vi "imp_test_v9_3.vi"() -> ()   [LabVIEW 2014]
uses:
  <vilib>/rvi/FXPMathLib/FxpSinAndCos/subVIs/nifxpmath_SinAndCos_SimConfig.ctl
  <vilib>/rvi/Emulation/niFpgaGetClockAttributes.vi
  <vilib>/rvi/Emulation/niFpgaSctlEmulationGetInTimedLoop.vi
  <vilib>/rvi/Emulation/niFpgaEmulationReportErrorSimple.vi
  <vilib>/rvi/Emulation/niFpgaProcessEmulError.vi
  <vilib>/rvi/interface/RandomDataEmulation/nirviRandomDataMultiElementFPGAFIFO.vi
  <instcachedir>/0/nirviRandomDataMultiElementFPGAFIFO_AD0CFC12EF974623A9C2E4184BC062B2.lvgen/nirviRandomDataMultiElementFPGAFIFO_AD0CFC12EF974623A9C2E4184BC062B2_025.vi
  <vilib>/rvi/interface/RandomDataEmulation/niFpgaRandomDataHandleErrors.vi
  <vilib>/rvi/Emulation/niFpgaCriticalErrorInLSC.vi
  <vilib>/rvi/FXPMathLib/FxpSinAndCos/simVIs/DllFxpSinAndCosTemp_sub.vi
  <vilib>/rvi/eio/common/nirviEmuTemplateMethod_errors.vi
  <vilib>/rvi/DataTransferAndStorage/Container/XNode/niFpgaContainer.xnode
  <vilib>/rvi/interface/RandomDataEmulation/nirviRandomDataFpgaMultiElementTemplate.vi
  <vilib>/rvi/FXPMathLib/FxpSinAndCos/XNode/nifxpmath_SinAndCos.xnode
  <vilib>/eio/EIONode/EIONode.xnode
  <vilib>/rvi/Analysis/measure/butterworth/XNode/niFpgaButterworthFilter.xnode
panel:
  out "Dpr_ramp":fxp<+/-,22,7>
  out "Dyr_ramp":fxp<+/-,22,7>
  in  "Dp_stroke (mm)":fxp<+/-,22,7>
  in  "Dy_stroke (mm)":fxp<+/-,22,7>
  in  "Vp (mm/s)":fxp<+/-,30,6>
  in  "Vy (mm/s)":fxp<+/-,30,6>
  out "omega_p (Mavg w. f)":fxp<+/-,36,18>
  in  "scaled coefficients":i32[](array[numeric])=[946630756, 63555534]
  in  "FIFO":i16(ring) items=["Pitch_F+P", "imp ctrl", "Yaw_F+P"]
  out "PID (kHz)":fxp<+/-,20,10>
  out "Dy1_d (T)":fxp<+/-,36,13>
  out "omega_y1 (T)":fxp<+/-,36,13>
  out "Dp1_d (T)":fxp<+/-,36,13>
  out "omega_p1 (T)":fxp<+/-,36,13>
  out "Dy2_d (T)":fxp<+/-,36,13>
  out "Dp2_d (T)":fxp<+/-,36,13>
  out "omega_y2 (T)":fxp<+/-,36,13>
  out "omega_p2 (T)":fxp<+/-,36,13>
  out "mt_omega_y2":u32
  out "mt_omega_p2":u32
  out "rad_y2":fxp<+/-,33,20>
  out "D_y2":fxp<+/-,32,7>
  out "rad_y1":fxp<+/-,33,20>
  out "D_y1":fxp<+/-,32,7>
  out "Encoder Position_y1":i32
  out "Encoder Position_y2":i32
  out "Encoder Position_p2":i32
  out "D_p2":fxp<+/-,32,7>
  out "rad_p2":fxp<+/-,33,20>
  out "D_p1":fxp<+/-,32,7>
  out "rad_p1":fxp<+/-,33,20>
  out "Encoder Position_p1":i32
  in  "Mag. factor_y":fxp<+/-,20,3>
  in  "Mag. encoder_y":bool
  out "omega_y (rad/s)":fxp<+/-,36,13>
  out "Dy_d (mm/s)":fxp<+/-,36,13>
  in  "Vy. Est.":i16(ring) items=["T", "Mavg"]
  out "omega_y (Mavg)":fxp<+/-,36,14>
  out "Dy_d (Mavg)":fxp<+/-,36,14>
  in  "Dy_d_M_avg_Tc (uSec)":i32
  out "Dp_d (Mavg)":fxp<+/-,36,14>
  out "omega_p (Mavg)":fxp<+/-,36,14>
  in  "Dp_d_M_avg_Tc (uSec)":i32
  out "Dp_d (T)":fxp<+/-,36,13>
  out "omega_p (T)":fxp<+/-,36,13>
  in  "Vp. Est.":i16(ring) items=["T", "Mavg"]
  in  "Mag. factor_p":fxp<+/-,20,3>
  in  "Mag. encoder_p":bool
  in  "Belt_out_p":fxp<+/-,7,7>
  in  "Belt_in_p":fxp<+/-,6,6>
  in  "Belt_out_y":fxp<+/-,7,7>
  in  "Belt_in_y":fxp<+/-,6,6>
  in  "mt0_omega_p":u32
  in  "Encoder reset":bool
  out "Dpr_sin":fxp<+/-,22,7>
  in  "Sin offset_p":fxp<+/-,22,7>
  in  "Sin magnitude_p":fxp<+/-,21,6>
  out "Dpr_sin_dd":fxp<+/-,35,20>
  out "Dpr_sin_d":fxp<+/-,33,15>
  out "Sin omega_p":fxp<+/-,34,9>
  in  "Sin wave freq._p (Hz)":fxp<+/-,32,6>
  in  "Dpr_step":fxp<+/-,22,7>
  out "Dpr_for":fxp<+/-,22,7>
  in  "Command_p":i16(ring) items=["Step", "Sine", "Ramp"]
  out "Fp_PID":fxp<+/-,36,16>
  in  "Kp_p":fxp<+/-,32,13>
  out "va_p":fxp<+/-,36,7>
  out "vb_p":fxp<+/-,37,8>
  out "vq_p_F":fxp<+/-,20,5> format="%.57g"
  out "vd_p_F":fxp<+/-,20,5>
  in  "Stop motor_p":bool
  out "Dp_d (mm/s)":fxp<+/-,36,13>
  out "omega_p (rad/s)":fxp<+/-,36,13>
  out "mt_omega_p1":u32
  out "rad_p(NrTheta)":fxp<+/-,33,20>
  out "D_p(mm)":fxp<+/-,32,7>
  out "Encoder Position_p":i32
  in  "Encoder reset_p":bool
  out "Dyr_for":fxp<+/-,22,7>
  in  "Command_y":i16(ring) items=["Step", "Sine", "Ramp"]
  out "vb_y":fxp<+/-,38,8>
  out "va_y":fxp<+/-,38,8>
  out "Dyr_sin_dd":fxp<+/-,35,20>
  out "Dyr_sin_d":fxp<+/-,33,15>
  out "Sin omega_y":fxp<+/-,34,9>
  out "Dyr_sin":fxp<+/-,22,7>
  in  "Sin offset_y":fxp<+/-,22,7>
  in  "Sin magnitude_y":fxp<+/-,21,6>
  out "Time now(s)":fxp<+,52,14>
  in  "Sin wave freq._y (Hz)":fxp<+/-,32,6>
  in  "Dyr_step":fxp<+/-,22,7>
  out "Fy_PID":fxp<+/-,36,16>
  in  "Kp_y":fxp<+/-,32,13>
  out "vq_y_F":fxp<+/-,20,5> format="%.57g"
  out "vd_y_F":fxp<+/-,20,5>
  in  "Stop motor_y":bool
  out "Dy_d (T)":fxp<+/-,36,13>
  out "omega_y (T)":fxp<+/-,36,13>
  in  "mt0_omega_y":u32
  out "mt_omega_y1":u32
  out "rad_y(NrTheta)":fxp<+/-,33,20>
  out "D_y(mm)":fxp<+/-,32,7>
  out "Encoder Position_y":i32
  in  "Encoder reset_y":bool
  in  "Ini coe.":bool
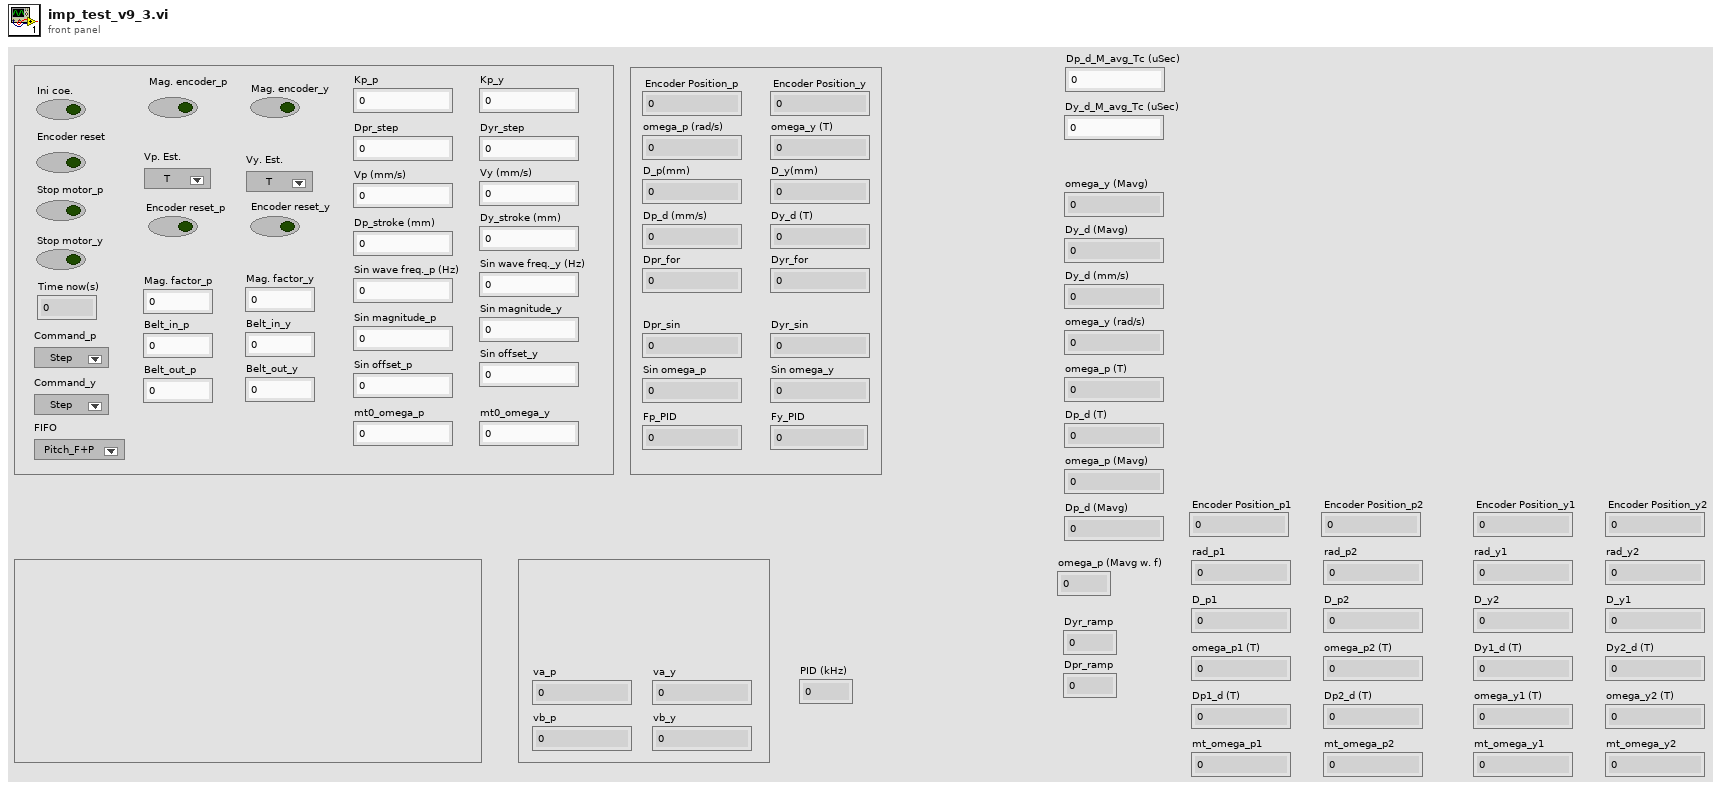
[diagram p1: front panel]
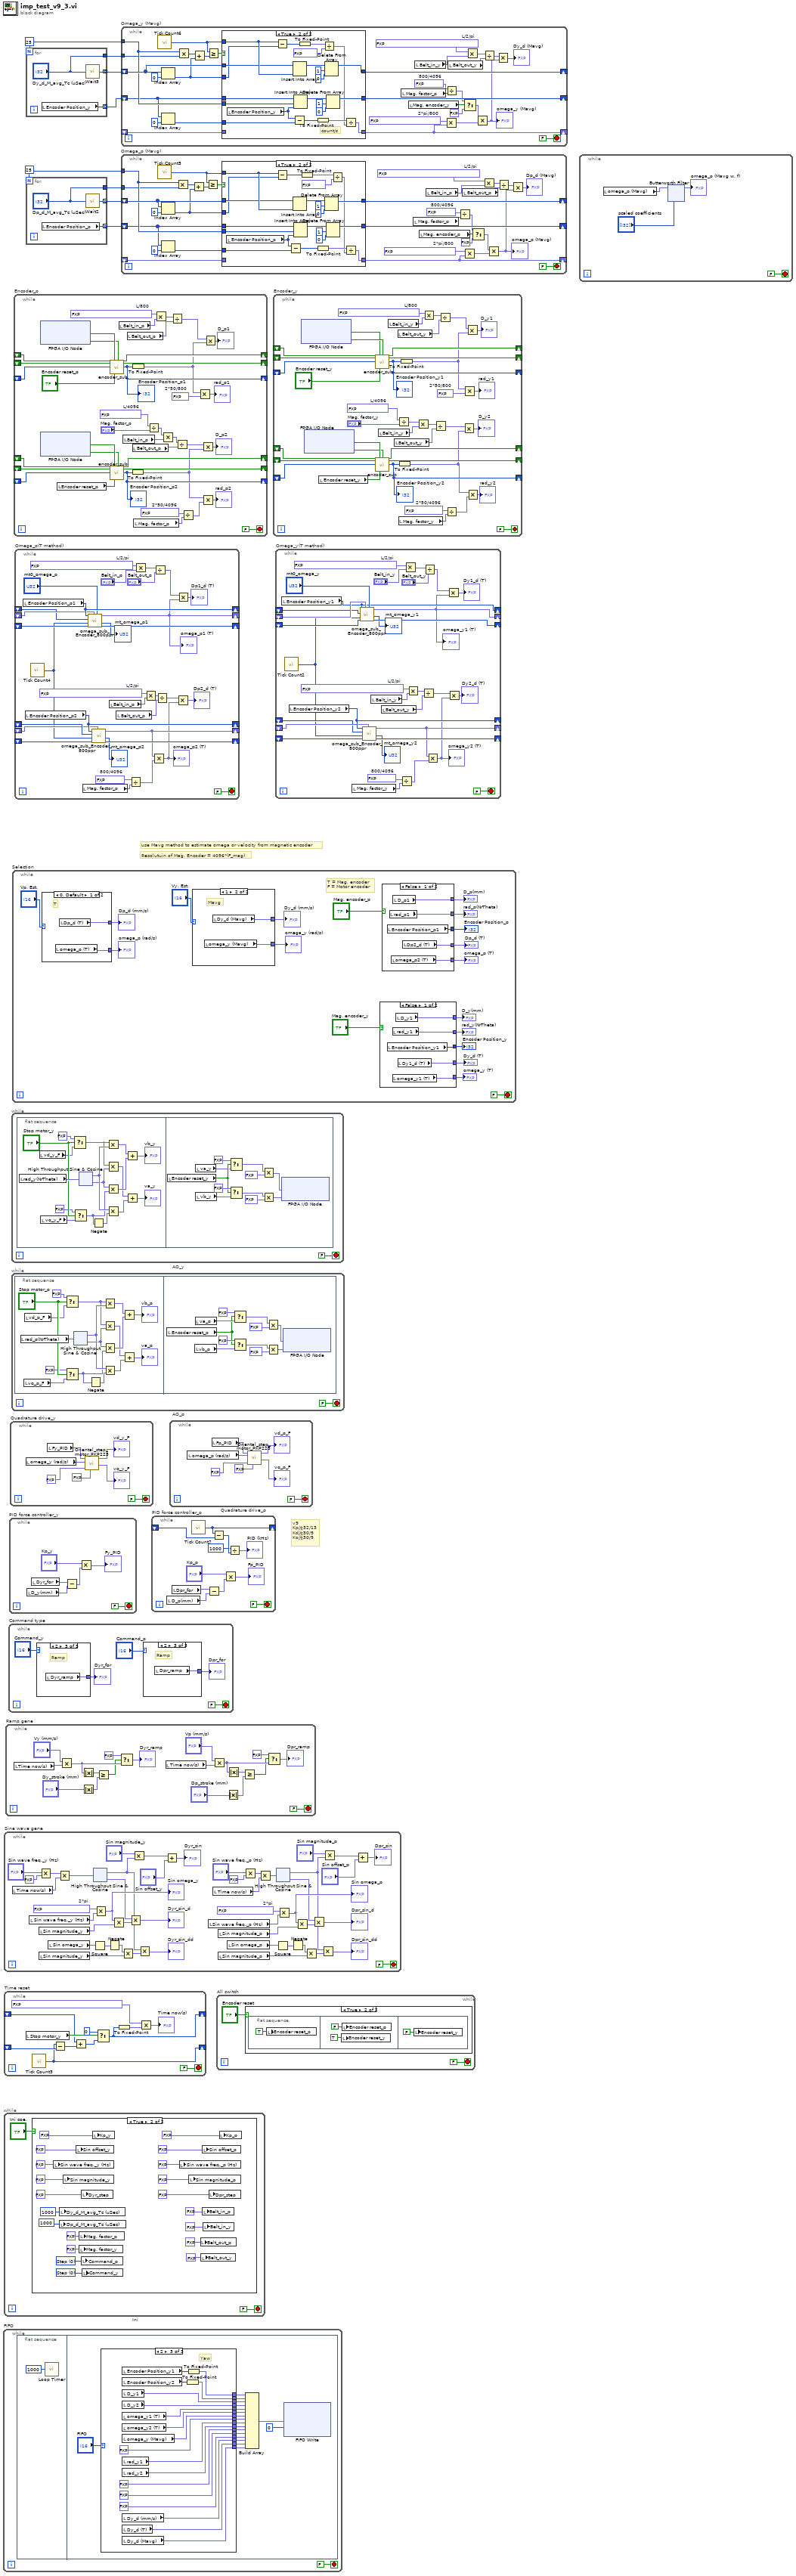
[diagram p0: block diagram]
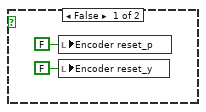
[diagram p4: hidden frame]
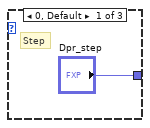
[diagram p5: hidden frame]
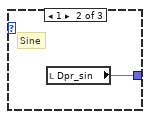
[diagram p6: hidden frame]
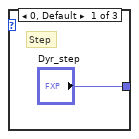
[diagram p7: hidden frame]
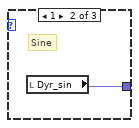
[diagram p8: hidden frame]
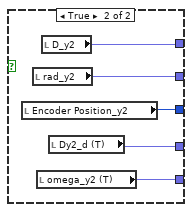
[diagram p9: hidden frame]
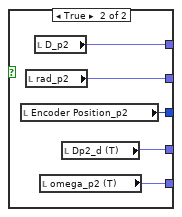
[diagram p10: hidden frame]
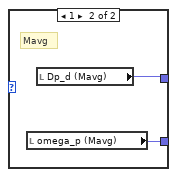
[diagram p11: hidden frame]
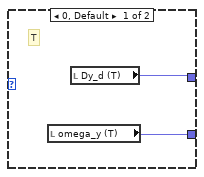
[diagram p12: hidden frame]
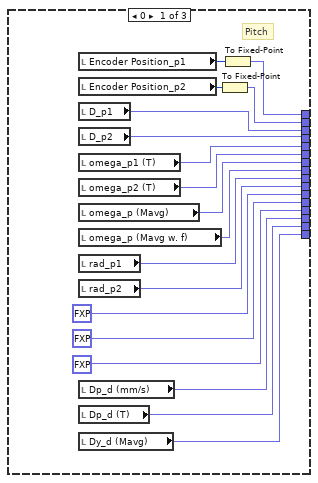
[diagram p14: hidden frame]
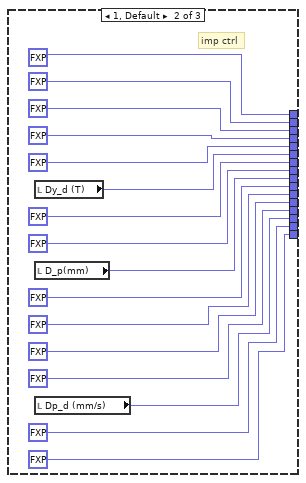
[diagram p15: hidden frame]
diagram:
  w5 = 25
  w8 = 25
  # "v9\nKp改32/13\nKd改30/9\nKo改30/9"
  # "Resolutuin of Mag. Encoder = 4096*(F_mag)"
  # "use Mavg method to estimate omega or velocity from magnetic encoder"
  n1 = while "FIFO" {
    stop <- FALSE stop-if-true
    n2 = flat-sequence {
      frame #0 {
        n3 = call "Loop Timer"("Count(uSec)"=u32 1000) -> ()  [unwired: 1 out]
      }
      frame #1 {
        n4 = case shown="2" "FIFO" {
          tunnel: [w30 fxp<+,1,1> 0.0 w64] -> w11
          tunnel: [w31 fxp<+,1,1> 0.0 w65] -> w29
          tunnel: [w47 fxp<+,1,1> 0.0 w81] -> w28
          tunnel: [w46 fxp<+,1,1> 0.0 w80] -> w27
          tunnel: [w43 fxp<+,1,1> 0.0 w77] -> w25
          tunnel: [w44 w63 w78] -> w24
          tunnel: [w45 fxp<+,1,1> 0.0 w79] -> w23
          tunnel: [w42 w62 w76] -> w22
          tunnel: [w41 fxp<+,1,1> 0.0 w75] -> w21
          tunnel: [fxp<+,1,1> 0.0 fxp<+,1,1> 0.0 fxp<+,1,1> 0.0] -> w20
          tunnel: [fxp<+,1,1> 0.0 fxp<+,1,1> 0.0 fxp<+,1,1> 0.0] -> w19
          tunnel: [fxp<+,1,1> 0.0 fxp<+,1,1> 0.0 fxp<+,1,1> 0.0] -> w18
          tunnel: [w40 w61 w74] -> w17
          tunnel: [w39 fxp<+,1,1> 0.0 w73] -> w16
          tunnel: [w34 fxp<+,1,1> 0.0 ("element") w72] -> w15
          tunnel: [w38 fxp<+,1,1> 0.0 fxp<+,1,1> 0.0] -> w13
          frame 0 {
            # "Pitch"
            n5 = local read "Encoder Position_p1"() -> (w33:i32)
            n6 = local read "Encoder Position_p2"() -> (w32:i32)
            n7 = local read "D_p1"() -> (w47:fxp<+/-,32,7>)
            n8 = local read "D_p2"() -> (w46:fxp<+/-,32,7>)
            n9 = local read "omega_p1 (T)"() -> (w45:fxp<+/-,36,13>)
            n10 = local read "omega_p2 (T)"() -> (w44:fxp<+/-,36,13>)
            n11 = local read "omega_p (Mavg)"() -> (w43:fxp<+/-,36,14>)
            n12 = local read "omega_p (Mavg w. f)"() -> (w38:fxp<+/-,36,18>)
            n13 = local read "rad_p1"() -> (w42:fxp<+/-,33,20>)
            n14 = local read "rad_p2"() -> (w41:fxp<+/-,33,20>)
            n15 = local read "Dp_d (mm/s)"() -> (w40:fxp<+/-,36,13>)
            n16 = local read "Dp_d (T)"() -> (w39:fxp<+/-,36,13>)
            n17 = local read "Dy_d (Mavg)"() -> (w34:fxp<+/-,36,14>)
            n18 = To Fixed-Point(number=w32) -> (fixed-point=w31:fxp<+/-,25,25>)  [unwired: 1 in]
            n19 = To Fixed-Point(number=w33) -> (fixed-point=w30:fxp<+/-,25,25>)  [unwired: 1 in]
          }
          frame 1, Default {
            # "imp ctrl"
            n20 = local read "Dy_d (T)"() -> (w63:fxp<+/-,36,13>)
            n21 = local read "D_p(mm)"() -> (w62:fxp<+/-,32,7>)
            n22 = local read "Dp_d (mm/s)"() -> (w61:fxp<+/-,36,13>)
          }
          frame 2 {
            # "Yaw"
            n23 = local read "Encoder Position_y1"() -> (w67:i32)
            n24 = local read "Encoder Position_y2"() -> (w66:i32)
            n25 = local read "D_y1"() -> (w81:fxp<+/-,32,7>)
            n26 = local read "D_y2"() -> (w80:fxp<+/-,32,7>)
            n27 = local read "omega_y1 (T)"() -> (w79:fxp<+/-,36,13>)
            n28 = local read "omega_y2 (T)"() -> (w78:fxp<+/-,36,13>)
            n29 = local read "omega_y (Mavg)"() -> (w77:fxp<+/-,36,14>)
            n30 = local read "rad_y1"() -> (w76:fxp<+/-,33,20>)
            n31 = local read "rad_y2"() -> (w75:fxp<+/-,33,20>)
            n32 = local read "Dy_d (mm/s)"() -> (w74:fxp<+/-,36,13>)
            n33 = local read "Dy_d (T)"() -> (w73:fxp<+/-,36,13>)
            n34 = local read "Dy_d (Mavg)"() -> (w72:fxp<+/-,36,14>)
            n35 = To Fixed-Point(number=w66) -> (fixed-point=w65:fxp<+/-,25,25>)  [unwired: 1 in]
            n36 = To Fixed-Point(number=w67) -> (fixed-point=w64:fxp<+/-,25,25>)  [unwired: 1 in]
          }
        }
        n37 = Build Array(w11, w29, w28, w27, w23, w24, w25, w13, w22, w21, w20, w19, w18, w17, w16, w15) -> (w14:fxp<+/-,50,25>[])
        n38 = xnode ("FIFO Write")("Element"=w14, "Timeout"=0) -> ()  [unwired: 1 in, 2 out]
      }
    }
  }
  n39 = while "Sine wave gene" {
    stop <- FALSE stop-if-true
    w87 = fxp<+,20,3> 6.2831878662109375  # 2*pi
    w119 = fxp<+,20,3> 6.2831878662109375  # 2*pi
    n40 = local read "Time now(s)"() -> (w125:fxp<+,52,14>)
    n41 = local read "Sin wave freq._y (Hz)"() -> (w118:fxp<+/-,32,6>)
    n42 = Multiply(x="Sin wave freq._y (Hz)", y=fxp<+/-,10,3> 2.0) -> (x*y=w126:fxp<+/-,41,9>)
    n43 = local read "Sin magnitude_y"() -> (w116:fxp<+/-,21,6>)
    n44 = local read "Sin magnitude_y"() -> (w109:fxp<+/-,21,6>)
    n45 = local read "Sin omega_y"() -> (w112:fxp<+/-,34,9>)
    n46 = Multiply(x=w126, y=w125) -> (x*y=w124:fxp<+/-,41,19>)
    n47 = Square(x=w112) -> (x^2=w111:fxp<+,34,18>)
    n48 = xnode "High Throughput Sine & Cosine"("x (pi)"=w124) -> ("sin(x)"=w106:fxp<+/-,16,2>, "cos(x)"=w114:fxp<+/-,16,2>)
    n49 = Multiply(x=w119, y=w118) -> (x*y=w117:fxp<+/-,34,9>)
    "Sin omega_y" <- w117
    n50 = Negate(x=w111) -> (-x=w110:fxp<+/-,35,19>)
    n51 = Multiply(x=w117, y=w116) -> (x*y=w115:fxp<+/-,33,15>)
    n52 = Multiply(x=w110, y=w109) -> (x*y=w108:fxp<+/-,34,20>)
    n53 = Multiply(x=w114, y=w115) -> (x*y=→"Dyr_sin_d":fxp<+/-,33,15>)
    n54 = Multiply(x="Sin magnitude_y", y=w106) -> (x*y=w122:fxp<+/-,37,8>)
    n55 = Multiply(x=w106, y=w108) -> (x*y=→"Dyr_sin_dd":fxp<+/-,35,20>)
    n56 = Add(x=w122, y="Sin offset_y") -> (x+y=→"Dyr_sin":fxp<+/-,37,8>)
    n57 = local read "Sin wave freq._p (Hz)"() -> (w83:fxp<+/-,32,6>)
    n58 = local read "Time now(s)"() -> (w101:fxp<+,52,14>)
    n59 = local read "Sin magnitude_p"() -> (w84:fxp<+/-,21,6>)
    n60 = local read "Sin magnitude_p"() -> (w86:fxp<+/-,21,6>)
    n61 = local read "Sin omega_p"() -> (w85:fxp<+/-,34,9>)
    n62 = Multiply(x="Sin wave freq._p (Hz)", y=fxp<+/-,10,3> 2.0) -> (x*y=w105:fxp<+/-,42,9>)
    n63 = Multiply(x=w105, y=w101) -> (x*y=w102:fxp<+/-,41,19>)
    n64 = Square(x=w85) -> (x^2=w97:fxp<+,34,18>)
    n65 = xnode "High Throughput Sine & Cosine"("x (pi)"=w102) -> ("sin(x)"=w88:fxp<+/-,16,2>, "cos(x)"=w93:fxp<+/-,16,2>)
    n66 = Multiply(x=w87, y=w83) -> (x*y=w100:fxp<+/-,34,9>)
    "Sin omega_p" <- w100
    n67 = Negate(x=w97) -> (-x=w96:fxp<+/-,35,19>)
    n68 = Multiply(x=w100, y=w84) -> (x*y=w99:fxp<+/-,33,15>)
    n69 = Multiply(x=w96, y=w86) -> (x*y=w95:fxp<+/-,35,19>)
    n70 = Multiply(x=w93, y=w99) -> (x*y=→"Dpr_sin_d":fxp<+/-,33,15>)
    n71 = Multiply(x=w88, y=w95) -> (x*y=→"Dpr_sin_dd":fxp<+/-,35,20>)
    n72 = Multiply(x="Sin magnitude_p", y=w88) -> (x*y=w91:fxp<+/-,37,8>)
    n73 = Add(x=w91, y="Sin offset_p") -> (x+y=→"Dpr_sin":fxp<+/-,37,8>)
  }
  n74 = while "Time reset" {
    shift-right: [w198] -> _
    shift-left: _ -> [w199]
    shift-right: [w193] -> _
    shift-left: _ -> [w194]
    stop <- FALSE stop-if-true
    n75 = local read "Stop motor_y"() -> (w200:bool)
    n76 = call "Tick Count3"() -> ("Tick Count(uSec)"=w198:u32)
    n77 = Subtract(x=w198, y=w199) -> (x-y=w197:u32)
    n78 = Add(x=w194, y=w197) -> (x+y=w196:u32)
    n79 = Select(t=u32 0, s=w200, f=w196) -> (s? t:f=w193:u32)
    n80 = To Fixed-Point(number=w193) -> (fixed-point=w192:fxp<+,32,32>)  [unwired: 1 in]
    n81 = Multiply(x=fxp<+,20,-18> 1.0000003385357559e-06, y=w192) -> (x*y=→"Time now(s)":fxp<+,52,14>)
  }
  n82 = while "Ini" {
    stop <- FALSE stop-if-true
    n83 = case shown="True" "Ini coe." {
      frame False {
      }
      frame True {
        w216 = i16 0 items=["Step", "Sine"] ("Command_p")
        w217 = i16 0 items=["Step", "Sine"] ("Command_y")
        n84 = local write "Sin wave freq._y (Hz)"(fxp<+/-,32,6> 1.0 ("Sin wave freq. (Hz)")) -> ()
        n85 = local write "Dp_d_M_avg_Tc (uSec)"(u32 1000 ("D_d_M_avg_Tc (uSec)")) -> ()
        n86 = local write "Dy_d_M_avg_Tc (uSec)"(1000 ("Dy_d_M_avg_Tc (uSec)")) -> ()
        n87 = local write "Sin magnitude_y"(fxp<+/-,22,7> 5.0 ("Sin magnitude")) -> ()
        n88 = local write "Sin offset_y"(fxp<+/-,38,9> 0.0 ("Sin offset")) -> ()
        n89 = local write "Mag. factor_p"(fxp<+/-,20,3> 1.0 ("Mag. factor_p")) -> ()
        n90 = local write "Mag. factor_y"(fxp<+/-,20,3> 1.0 ("Mag. factor_y")) -> ()
        n91 = local write "Command_p"(w216) -> ()
        n92 = local write "Dyr_step"(fxp<+/-,22,7> 0.0 ("Dr")) -> ()
        n93 = local write "Command_y"(w217) -> ()
        n94 = local write "Kp_y"(fxp<+/-,36,9> 30.0 ("Kp")) -> ()
        n95 = local write "Sin wave freq._p (Hz)"(fxp<+/-,32,6> 1.0 ("Sin wave freq._p (Hz)")) -> ()
        n96 = local write "Sin magnitude_p"(fxp<+/-,21,6> 5.0 ("Sin magnitude_p")) -> ()
        n97 = local write "Belt_out_p"(fxp<+/-,7,7> 22.0 ("Belt_op")) -> ()
        n98 = local write "Belt_out_y"(fxp<+/-,7,7> 22.0 ("Belt_oy")) -> ()
        n99 = local write "Sin offset_p"(fxp<+/-,22,7> 0.0 ("Sin offset_p")) -> ()
        n100 = local write "Belt_in_p"(fxp<+/-,6,6> 16.0 ("Belt_mp")) -> ()
        n101 = local write "Belt_in_y"(fxp<+/-,6,6> 16.0 ("Belt_my")) -> ()
        n102 = local write "Dpr_step"(fxp<+/-,22,7> 0.0 ("Dpr_step")) -> ()
        n103 = local write "Kp_p"(fxp<+/-,36,9> 30.0 ("Kp_p")) -> ()
      }
    }
  }
  n104 = while "Ramp gene" {
    stop <- FALSE stop-if-true
    n105 = local read "Time now(s)"() -> (w240:fxp<+,52,14>)
    n106 = Multiply(x="Vy (mm/s)", y=w240) -> (x*y=w229:fxp<+/-,64,20>)
    n107 = Absolute Value(x=w229) -> (abs(x)=w237:fxp<+,64,20>)
    n108 = Absolute Value(x="Dy_stroke (mm)") -> (abs(x)=w236:fxp<+,22,7>)
    n109 = Greater Or Equal?(x=w237, y=w236) -> (x >= y?=w228:bool)
    n110 = Select(t=fxp<+,1,1> 0.0, s=w228, f=w229) -> (s? t:f=→"Dyr_ramp":fxp<+/-,64,20>)
    n111 = local read "Time now(s)"() -> (w238:fxp<+,52,14>)
    n112 = Multiply(x="Vp (mm/s)", y=w238) -> (x*y=w227:fxp<+/-,64,20>)
    n113 = Absolute Value(x="Dp_stroke (mm)") -> (abs(x)=w233:fxp<+,22,7>)
    n114 = Absolute Value(x=w227) -> (abs(x)=w234:fxp<+,64,20>)
    n115 = Greater Or Equal?(x=w234, y=w233) -> (x >= y?=w226:bool)
    n116 = Select(t=fxp<+,1,1> 0.0, s=w226, f=w227) -> (s? t:f=→"Dpr_ramp":fxp<+/-,64,20>)
  }
  n117 = while "Command type" {
    stop <- FALSE stop-if-true
    n118 = case shown="2" "Command_y" {
      tunnel: ["Dyr_step" w251 w252] -> w245
      frame 0, Default {
        # "Step"
      }
      frame 1 {
        # "Sine"
        n119 = local read "Dyr_sin"() -> (w251:fxp<+/-,22,7>)
      }
      frame 2 {
        # "Ramp"
        n120 = local read "Dyr_ramp"() -> (w252:fxp<+/-,22,7>)
      }
    }
    "Dyr_for" <- w245
    n121 = case shown="2" "Command_p" {
      tunnel: ["Dpr_step" w248 w249] -> w243
      frame 0, Default {
        # "Step"
      }
      frame 1 {
        # "Sine"
        n122 = local read "Dpr_sin"() -> (w248:fxp<+/-,22,7>)
      }
      frame 2 {
        # "Ramp"
        n123 = local read "Dpr_ramp"() -> (w249:fxp<+/-,22,7>)
      }
    }
    "Dpr_for" <- w243
  }
  n124 = while "PID force controller_y" {
    stop <- FALSE stop-if-true
    n125 = local read "D_y(mm)"() -> (w256:fxp<+/-,32,7>)
    n126 = local read "Dyr_for"() -> (w257:fxp<+/-,22,7>)
    n127 = Subtract(x=w257, y=w256) -> (x-y=w255:fxp<+/-,33,8>)
    n128 = Multiply(x="Kp_y", y=w255) -> (x*y=→"Fy_PID":fxp<+/-,64,20>)
  }
  n129 = while "Quadrature drive_y" {
    stop <- FALSE stop-if-true
    n130 = local read "omega_y (rad/s)"() -> (w265:fxp<+/-,36,13>)
    n131 = local read "Fy_PID"() -> (w261:fxp<+/-,36,16>)
    n132 = call "Oriental_step_motor_PKP225.vi"("F_Threshold"=fxp<+,12,12> 10.0, "dFmr"=fxp<+,1,1> 0.0 ("f"), "omega"=w265, "Fmr"=w261) -> ("vq_F"=→"vq_y_F":fxp<+/-,20,5>, "vd_F"=→"vd_y_F":fxp<+/-,20,5>)  [unwired: 6 in]
  }
  n133 = while "AO_p" {
    stop <- FALSE stop-if-true
    n134 = flat-sequence {
      frame #0 {
        n135 = local read "rad_p(NrTheta)"() -> (w278:fxp<+/-,33,20>)
        n136 = local read "vq_p_F"() -> (w279:fxp<+/-,20,5>)
        n137 = local read "vd_p_F"() -> (w281:fxp<+/-,20,5>)
        n138 = Select(t=fxp<+/-,20,5> 0.0, s="Stop motor_p", f=w281) -> (s? t:f=w270:fxp<+/-,20,5>)
        n139 = Select(t=fxp<+,1,1> 0.0, s="Stop motor_p", f=w279) -> (s? t:f=w269:fxp<+/-,20,5>)
        n140 = xnode "High Throughput Sine & Cosine"("x (pi)"=w278) -> ("sin(x)"=w272:fxp<+/-,16,2>, "cos(x)"=w271:fxp<+/-,16,2>)
        n141 = Negate(x=w269) -> (-x=w277:fxp<+/-,21,6>)
        n142 = Multiply(x=w270, y=w272) -> (x*y=w276:fxp<+/-,36,7>)
        n143 = Multiply(x=w270, y=w271) -> (x*y=w274:fxp<+/-,36,7>)
        n144 = Multiply(x=w271, y=w269) -> (x*y=w275:fxp<+/-,36,7>)
        n145 = Multiply(x=w272, y=w277) -> (x*y=w273:fxp<+/-,35,6>)
        n146 = Add(x=w276, y=w275) -> (x+y=→"vb_p":fxp<+/-,37,8>)
        n147 = Add(x=w274, y=w273) -> (x+y=→"va_p":fxp<+/-,36,7>)
      }
      frame #1 {
        n148 = local read "Encoder reset_p"() -> (w314:bool)
        n149 = local read "vb_p"() -> (w315:fxp<+/-,37,8>)
        n150 = local read "va_p"() -> (w316:fxp<+/-,36,7>)
        n151 = Select(t=fxp<+,2,2> 3.0, s=w314, f=w316) -> (s? t:f=w322:fxp<+/-,36,7>)
        n152 = Select(t=fxp<+,1,1> 0.0, s=w314, f=w315) -> (s? t:f=w321:fxp<+/-,37,8>)
        n153 = Multiply(x=w322, y=fxp<+/-,1,0> -0.5) -> (x*y=w317:fxp<+/-,36,6>)
        n154 = Multiply(x=w321, y=fxp<+/-,1,0> -0.5) -> (x*y=w318:fxp<+/-,36,6>)
        n155 = xnode "FPGA I/O Node"("Mod8/AO0"=w317, "Mod8/AO1"=w318) -> ()  [unwired: 2 in, 2 out]
      }
    }
  }
  n156 = while "AO_y" {
    stop <- FALSE stop-if-true
    n157 = flat-sequence {
      frame #0 {
        n158 = local read "rad_y(NrTheta)"() -> (w342:fxp<+/-,33,20>)
        n159 = local read "vd_y_F"() -> (w340:fxp<+/-,20,5>)
        n160 = local read "vq_y_F"() -> (w339:fxp<+/-,20,5>)
        n161 = Select(t=fxp<+/-,20,5> 0.0, s="Stop motor_y", f=w340) -> (s? t:f=w334:fxp<+/-,20,5>)
        n162 = Select(t=fxp<+/-,20,5> 0.0, s="Stop motor_y", f=w339) -> (s? t:f=w333:fxp<+/-,20,5>)
        n163 = xnode "High Throughput Sine & Cosine"("x (pi)"=w342) -> ("sin(x)"=w336:fxp<+/-,17,2>, "cos(x)"=w335:fxp<+/-,17,2>)
        n164 = Negate(x=w333) -> (-x=w332:fxp<+/-,21,6>)
        n165 = Multiply(x=w334, y=w336) -> (x*y=w331:fxp<+/-,37,7>)
        n166 = Multiply(x=w334, y=w335) -> (x*y=w329:fxp<+/-,37,7>)
        n167 = Multiply(x=w335, y=w333) -> (x*y=w330:fxp<+/-,37,7>)
        n168 = Multiply(x=w336, y=w332) -> (x*y=w328:fxp<+/-,36,6>)
        n169 = Add(x=w331, y=w330) -> (x+y=→"vb_y":fxp<+/-,38,8>)
        n170 = Add(x=w329, y=w328) -> (x+y=→"va_y":fxp<+/-,37,7>)
      }
      frame #1 {
        n171 = local read "Encoder reset_y"() -> (w375:bool)
        n172 = local read "va_y"() -> (w374:fxp<+/-,38,8>)
        n173 = local read "vb_y"() -> (w373:fxp<+/-,38,8>)
        n174 = Select(t=fxp<+,2,2> 3.0, s=w375, f=w374) -> (s? t:f=w379:fxp<+/-,38,8>)
        n175 = Select(t=fxp<+,1,1> 0.0, s=w375, f=w373) -> (s? t:f=w378:fxp<+/-,38,8>)
        n176 = Multiply(x=w379, y=fxp<+/-,1,0> -0.5) -> (x*y=w382:fxp<+/-,39,8>)
        n177 = Multiply(x=w378, y=fxp<+/-,1,0> -0.5) -> (x*y=w383:fxp<+/-,37,6>)
        n178 = xnode "FPGA I/O Node"("Mod8/AO2"=w382, "Mod8/AO3"=w383) -> ()  [unwired: 2 in, 2 out]
      }
    }
  }
  n179 = while "Selection" {
    stop <- FALSE stop-if-true
    # "T = Mag. encoder\nF = Motor encoder"
    n180 = case shown="0, Default" "Vp. Est." {
      tunnel: [w424 w425] -> w398
      tunnel: [w423 w426] -> w399
      frame 0, Default {
        # "T"
        n181 = local read "omega_p (T)"() -> (w424:fxp<+/-,36,13>)
        n182 = local read "Dp_d (T)"() -> (w423:fxp<+/-,36,13>)
      }
      frame 1 {
        # "Mavg"
        n183 = local read "omega_p (Mavg)"() -> (w425:fxp<+/-,36,14>)
        n184 = local read "Dp_d (Mavg)"() -> (w426:fxp<+/-,36,14>)
      }
    }
    "Dp_d (mm/s)" <- w399
    "omega_p (rad/s)" <- w398
    n185 = case shown="1" "Vy. Est." {
      tunnel: [w428 w430] -> w401
      tunnel: [w427 w429] -> w402
      frame 0, Default {
        # "T"
        n186 = local read "omega_y (T)"() -> (w427:fxp<+/-,36,13>)
        n187 = local read "Dy_d (T)"() -> (w428:fxp<+/-,36,13>)
      }
      frame 1 {
        # "Mavg"
        n188 = local read "omega_y (Mavg)"() -> (w429:fxp<+/-,36,14>)
        n189 = local read "Dy_d (Mavg)"() -> (w430:fxp<+/-,36,14>)
      }
    }
    "Dy_d (mm/s)" <- w401
    "omega_y (rad/s)" <- w402
    n190 = case shown="False" "Mag. encoder_y" {
      tunnel: [w407 w411] -> w389
      tunnel: [w406 w412] -> w390
      tunnel: [w405 w410] -> w392
      tunnel: [w403 w409] -> w386
      tunnel: [w404 w408] -> w385
      frame False {
        n191 = local read "Encoder Position_y1"() -> (w405:i32)
        n192 = local read "rad_y1"() -> (w407:fxp<+/-,33,20>)
        n193 = local read "omega_y1 (T)"() -> (w403:fxp<+/-,36,13>)
        n194 = local read "D_y1"() -> (w406:fxp<+/-,32,7>)
        n195 = local read "Dy1_d (T)"() -> (w404:fxp<+/-,36,13>)
      }
      frame True {
        n196 = local read "Encoder Position_y2"() -> (w410:i32)
        n197 = local read "rad_y2"() -> (w411:fxp<+/-,33,20>)
        n198 = local read "omega_y2 (T)"() -> (w409:fxp<+/-,36,13>)
        n199 = local read "D_y2"() -> (w412:fxp<+/-,32,7>)
        n200 = local read "Dy2_d (T)"() -> (w408:fxp<+/-,36,13>)
      }
    }
    "D_y(mm)" <- w390
    "rad_y(NrTheta)" <- w389
    "Encoder Position_y" <- w392
    "Dy_d (T)" <- w385
    "omega_y (T)" <- w386
    n201 = case shown="False" "Mag. encoder_p" {
      tunnel: [w417 w422] -> w394
      tunnel: [w416 w421] -> w395
      tunnel: [w415 w420] -> w396
      tunnel: [w413 w419] -> w388
      tunnel: [w414 w418] -> w387
      frame False {
        n202 = local read "Encoder Position_p1"() -> (w415:i32)
        n203 = local read "rad_p1"() -> (w416:fxp<+/-,33,20>)
        n204 = local read "omega_p2 (T)"() -> (w413:fxp<+/-,36,13>)
        n205 = local read "D_p1"() -> (w417:fxp<+/-,32,7>)
        n206 = local read "Dp2_d (T)"() -> (w414:fxp<+/-,36,13>)
      }
      frame True {
        n207 = local read "Encoder Position_p2"() -> (w420:i32)
        n208 = local read "rad_p2"() -> (w421:fxp<+/-,33,20>)
        n209 = local read "D_p2"() -> (w422:fxp<+/-,32,7>)
        n210 = local read "omega_p2 (T)"() -> (w419:fxp<+/-,36,13>)
        n211 = local read "Dp2_d (T)"() -> (w418:fxp<+/-,36,13>)
      }
    }
    "D_p(mm)" <- w394
    "rad_p(NrTheta)" <- w395
    "Encoder Position_p" <- w396
    "Dp_d (T)" <- w387
    "omega_p (T)" <- w388
  }
  n212 = while "Encoder_p" {
    shift-right: [w468] -> _
    shift-left: _ -> [w467]
    shift-right: [w469] -> _
    shift-left: _ -> [w466]
    shift-right: [w463] -> _
    shift-left: _ -> [w465]
    shift-right: [w454] -> _
    shift-left: _ -> [w453]
    shift-right: [w455] -> _
    shift-left: _ -> [w456]
    shift-right: [w450] -> _
    shift-left: _ -> [w451]
    stop <- FALSE stop-if-true
    w446 = fxp<+/-,20,-5> 0.00048828125  # L/4096
    w444 = fxp<+/-,16,1> 0.0244140625  # 2*50/4096
    w462 = fxp<+/-,20,-5> 0.002499997615814209  # L/800
    w436 = fxp<+/-,16,1> 0.125  # 2*50/800
    n213 = xnode "FPGA I/O Node"() -> ("Mod7/DIO0"=w471:bool, "Mod7/DIO1"=w470:bool)  [unwired: 2 in, 2 out]
    n214 = xnode "FPGA I/O Node"() -> ("Mod7/DIO4"=w458:bool, "Mod7/DIO5"=w457:bool)  [unwired: 2 in, 2 out]
    n215 = local read "Encoder reset_p"() -> (w452:bool)
    n216 = call "encoder_sub.vi"("A_pre"=w467, "B_pre"=w466, "Encoder Position_pre"=w465, "A input"=w471, "Encoder Position Reset"="Encoder reset_p", "B input"=w470) -> ("A"=w468:bool, "B"=w469:bool, "Encoder Position (Counts)"=w463:i32)  [unwired: 19 in]
    "Encoder Position_p1" <- w463
    n217 = call "encoder_sub.vi"("A_pre"=w453, "B_pre"=w456, "Encoder Position_pre"=w451, "A input"=w458, "Encoder Position Reset"=w452, "B input"=w457) -> ("A"=w454:bool, "B"=w455:bool, "Encoder Position (Counts)"=w450:i32)  [unwired: 19 in]
    "Encoder Position_p2" <- w450
    n218 = local read "Belt_in_p"() -> (w461:fxp<+/-,6,6>)
    n219 = local read "Belt_in_p"() -> (w447:fxp<+/-,6,6>)
    n220 = local read "Belt_out_p"() -> (w459:fxp<+/-,7,7>)
    n221 = To Fixed-Point(number=w450) -> (fixed-point=w432:fxp<+/-,32,32>)  [unwired: 1 in]
    n222 = To Fixed-Point(number=w463) -> (fixed-point=w437:fxp<+/-,32,32>)  [unwired: 1 in]
    n223 = local read "Belt_out_p"() -> (w449:fxp<+/-,7,7>)
    n224 = local read "Mag. factor_p"() -> (w443:fxp<+/-,20,3>)
    n225 = Divide(x=w446, y="Mag. factor_p") -> (x/y=w445:fxp<+/-,41,13>)
    n226 = Multiply(x=w462, y=w461) -> (x*y=w460:fxp<+/-,26,1>)
    n227 = Multiply(x=w445, y=w447) -> (x*y=w448:fxp<+/-,46,18>)
    n228 = Divide(x=w460, y=w459) -> (x/y=w439:fxp<+/-,33,1>)
    n229 = Divide(x=w448, y=w449) -> (x/y=w434:fxp<+/-,53,18>)
    n230 = Divide(x=w444, y=w443) -> (x/y=w431:fxp<+/-,32,1>)
    n231 = Multiply(x=w437, y=w436) -> (x*y=→"rad_p1":fxp<+/-,33,20>)
    n232 = Multiply(x=w434, y=w432) -> (x*y=→"D_p2":fxp<+/-,37,7>)
    n233 = Multiply(x=w432, y=w431) -> (x*y=→"rad_p2":fxp<+/-,33,20>)
    n234 = Multiply(x=w439, y=w437) -> (x*y=→"D_p1":fxp<+/-,32,7>)
  }
  n235 = while "Omega_p(T method)" {
    shift-right: [w504] -> _
    shift-left: _ -> [w502]
    shift-right: [w475] -> _
    shift-left: _ -> [w503]
    shift-right: [w500] -> _
    shift-left: _ -> [w501]
    shift-right: [w491] -> _
    shift-left: _ -> [w490]
    shift-right: [w484] -> _
    shift-left: _ -> [w489]
    shift-right: [w488] -> _
    shift-left: _ -> [w487]
    stop <- FALSE stop-if-true
    w482 = fxp<+/-,32,0> 0.3183098859153688  # L/2/pi
    w493 = fxp<+,32,0> 0.1953125  # 800/4096
    w497 = fxp<+/-,32,0> 0.3183098859153688  # L/2/pi
    n236 = local read "Encoder Position_p1"() -> (w504:i32)
    n237 = local read "Encoder Position_p2"() -> (w491:i32)
    n238 = call "Tick Count4"() -> ("Tick Count(Ticks)"=w486:u32)
    n239 = local read "Mag. factor_p"() -> (w492:fxp<+/-,20,3>)
    n240 = call "omega_sub_Encoder_800ppr.vi"("mt0"="mt0_omega_p", "omega_pre"=w503, "ticks_m_pre"=w501, "ticks"=w486, "count_pre"=w502, "count"=w504) -> ("ticks_m"=w500:u32, "mt"=→"mt_omega_p1":u32, "omega"=w475:fxp<+/-,36,13>)  [unwired: 3 in]
    "omega_p1 (T)" <- w475
    n241 = call "omega_sub_Encoder_800ppr.vi"("omega_pre"=w489, "ticks_m_pre"=w487, "ticks"=w486, "count_pre"=w490, "count"=w491) -> ("ticks_m"=w488:u32, "mt"=→"mt_omega_p2":u32, "omega"=w484:fxp<+/-,36,13>)  [unwired: 4 in]
    n242 = local read "Belt_in_p"() -> (w480:fxp<+/-,6,6>)
    n243 = local read "Belt_out_p"() -> (w479:fxp<+/-,7,7>)
    n244 = Divide(x=w493, y=w492) -> (x/y=w483:fxp<+/-,32,1>)
    n245 = Multiply(x=w497, y="Belt_in_p") -> (x*y=w495:fxp<+/-,38,6>)
    n246 = Multiply(x=w482, y=w480) -> (x*y=w481:fxp<+/-,38,6>)
    n247 = Multiply(x=w484, y=w483) -> (x*y=w473:fxp<+/-,36,13>)
    "omega_p2 (T)" <- w473
    n248 = Divide(x=w495, y="Belt_out_p") -> (x/y=w476:fxp<+/-,20,1>)
    n249 = Divide(x=w481, y=w479) -> (x/y=w474:fxp<+/-,45,6>)
    n250 = Multiply(x=w474, y=w473) -> (x*y=→"Dp2_d (T)":fxp<+/-,36,13>)
    n251 = Multiply(x=w476, y=w475) -> (x*y=→"Dp1_d (T)":fxp<+/-,36,13>)
  }
  n252 = for {
    N: w5 -> [_]
    tunnel: [w507] -> w4 mode=indexing
    tunnel: [w506] -> w3 mode=indexing
    tunnel: ["Dy_d_M_avg_Tc (uSec)"] -> w2
    n253 = local read "Encoder Position_y"() -> (w506:i32)
    n254 = call "Wait3"("Count(uSec)"="Dy_d_M_avg_Tc (uSec)") -> ("Tick Count(uSec)"=w507:u32)
  }
  n255 = for {
    N: w8 -> [_]
    tunnel: ["Dp_d_M_avg_Tc (uSec)"] -> w1
    tunnel: [w509] -> w7 mode=indexing
    tunnel: [w508] -> w6 mode=indexing
    n256 = local read "Encoder Position_p"() -> (w508:i32)
    n257 = call "Wait2"("Count(uSec)"="Dp_d_M_avg_Tc (uSec)") -> ("Tick Count(uSec)"=w509:u32)
  }
  n258 = while "Omega_y (Mavg)" {
    tunnel: w5 -> [w534]
    shift-right: [w532] -> _
    shift-left: w4 -> [w537]
    shift-right: [w531] -> _
    shift-left: w3 -> [w533]
    shift-right: [w526] -> _
    shift-left: _ -> [w530]
    tunnel: w2 -> [w525]
    stop <- FALSE stop-if-true
    w513 = fxp<+/-,32,0> 0.3183098859153688  # L/2/pi
    w522 = fxp<+,32,0> 0.1953125  # 800/4096
    w528 = fxp<+/-,27,3> 0.007853984832763672  # 2*pi/800
    n259 = call "Tick Count6"() -> ("Tick Count(uSec)"=w538:u32)
    n260 = Index Array(array=w537, index=0) -> (element=w536:u32)
    n261 = Index Array(array=w533, index=0) -> (element=w535:i32)
    n262 = Multiply(x=w534, y=w525) -> (x*y=w540:i32)
    n263 = Add(x=w540, y=w536) -> (x+y=w539:u32)
    n264 = Greater Or Equal?(x=w538, y=w539) -> (x >= y?=w529:bool)
    n265 = case shown="True" w529 {
      tunnel: w538 -> [_ w561]
      tunnel: w534 -> [_ w558]
      tunnel: w537 -> [w545 w560]
      tunnel: w536 -> [_ w559]
      tunnel: w535 -> [_ w555]
      tunnel: w533 -> [w544 w557]
      tunnel: [w543 w553] -> w526
      tunnel: [w545 w552] -> w532
      tunnel: [w544 w551] -> w531
      tunnel: w530 -> [w543 _]
      frame False {
      }
      frame True {
        # "count/s"
        n266 = local read "Encoder Position_y"() -> (w554:i32)
        n267 = Subtract(x=w561, y=w559) -> (x-y=w562:u32)
        n268 = Insert Into Array(array=w560, new element=w561) -> (w564:u32[])  [unwired: 1 in]
        n269 = Subtract(x=w554, y=w555) -> (x-y=w549:i32)
        n270 = Insert Into Array(array=w557, index=w558, new element=w554) -> (w565:i32[])
        n271 = To Fixed-Point(number=w562) -> (fixed-point=w548:fxp<+,32,32>)  [unwired: 1 in]
        n272 = To Fixed-Point(number=w549) -> (fixed-point=w556:fxp<+/-,32,32>)  [unwired: 1 in]
        n273 = Divide(x=w548, y=fxp<+,32,32> 1000000.0) -> (x/y=w547:fxp<+/-,64,32>)
        n274 = Delete From Array(array=w564, length=1, index=0) -> (array with subset deleted=w552:u32[])  [unwired: 1 out]
        n275 = Delete From Array(array=w565, length=1, index=0) -> (array with subset deleted=w551:i32[])  [unwired: 1 out]
        n276 = Divide(x=w556, y=w547) -> (x/y=w553:fxp<+/-,40,20>)
      }
    }
    n277 = local read "Mag. factor_p"() -> (w521:fxp<+/-,20,3>)
    n278 = local read "Mag. encoder_y"() -> (w524:bool)
    n279 = local read "Belt_in_y"() -> (w515:fxp<+/-,6,6>)
    n280 = Multiply(x=w528, y=w526) -> (x*y=w518:fxp<+/-,44,14>)
    n281 = Divide(x=w522, y=w521) -> (x/y=w520:fxp<+/-,32,1>)
    n282 = local read "Belt_out_y"() -> (w516:fxp<+/-,7,7>)
    n283 = Select(t=w520, s=w524, f=fxp<+/-,2,2> 1.0) -> (s? t:f=w519:fxp<+/-,33,2>)
    n284 = Multiply(x=w513, y=w515) -> (x*y=w514:fxp<+/-,38,6>)
    n285 = Multiply(x=w519, y=w518) -> (x*y=w517:fxp<+/-,36,14>)
    "omega_y (Mavg)" <- w517
    n286 = Divide(x=w514, y=w516) -> (x/y=w512:fxp<+/-,45,6>)
    n287 = Multiply(x=w512, y=w517) -> (x*y=→"Dy_d (Mavg)":fxp<+/-,36,14>)
  }
  n288 = while "Omega_p (Mavg)" {
    tunnel: w8 -> [w591]
    shift-right: [w589] -> _
    shift-left: w7 -> [w594]
    shift-right: [w588] -> _
    shift-left: w6 -> [w590]
    shift-right: [w587] -> _
    shift-left: _ -> [w586]
    tunnel: w1 -> [w584]
    stop <- FALSE stop-if-true
    w573 = fxp<+/-,27,3> 0.007853984832763672  # 2*pi/800
    w575 = fxp<+,32,0> 0.1953125  # 800/4096
    w572 = fxp<+/-,32,0> 0.3183098859153688  # L/2/pi
    n289 = call "Tick Count5"() -> ("Tick Count(uSec)"=w595:u32)
    n290 = Index Array(array=w594, index=0) -> (element=w593:u32)
    n291 = Index Array(array=w590, index=0) -> (element=w592:i32)
    n292 = Multiply(x=w591, y=w584) -> (x*y=w597:i32)
    n293 = Add(x=w597, y=w593) -> (x+y=w596:u32)
    n294 = Greater Or Equal?(x=w595, y=w596) -> (x >= y?=w585:bool)
    n295 = case shown="True" w585 {
      tunnel: w595 -> [_ w618]
      tunnel: w591 -> [_ w615]
      tunnel: w594 -> [w602 w617]
      tunnel: w593 -> [_ w616]
      tunnel: w592 -> [_ w612]
      tunnel: w590 -> [w601 w614]
      tunnel: [w600 w610] -> w587
      tunnel: [w602 w609] -> w589
      tunnel: [w601 w608] -> w588
      tunnel: w586 -> [w600 _]
      frame False {
      }
      frame True {
        n296 = local read "Encoder Position_p"() -> (w611:i32)
        n297 = Subtract(x=w618, y=w616) -> (x-y=w619:u32)
        n298 = Subtract(x=w611, y=w612) -> (x-y=w603:i32)
        n299 = Insert Into Array(array=w617, new element=w618) -> (w621:u32[])  [unwired: 1 in]
        n300 = Insert Into Array(array=w614, index=w615, new element=w611) -> (w622:i32[])
        n301 = To Fixed-Point(number=w619) -> (fixed-point=w605:fxp<+,32,32>)  [unwired: 1 in]
        n302 = To Fixed-Point(number=w603) -> (fixed-point=w613:fxp<+/-,32,32>)  [unwired: 1 in]
        n303 = Delete From Array(array=w621, length=1, index=0) -> (array with subset deleted=w609:u32[])  [unwired: 1 out]
        n304 = Delete From Array(array=w622, length=1, index=0) -> (array with subset deleted=w608:i32[])  [unwired: 1 out]
        n305 = Divide(x=w605, y=fxp<+,32,32> 1000000.0) -> (x/y=w606:fxp<+/-,64,32>)
        n306 = Divide(x=w613, y=w606) -> (x/y=w610:fxp<+/-,40,20>)
      }
    }
    n307 = local read "Mag. factor_p"() -> (w576:fxp<+/-,20,3>)
    n308 = local read "Mag. encoder_p"() -> (w583:bool)
    n309 = local read "Belt_in_p"() -> (w580:fxp<+/-,6,6>)
    n310 = Divide(x=w575, y=w576) -> (x/y=w574:fxp<+/-,32,1>)
    n311 = local read "Belt_out_p"() -> (w579:fxp<+/-,7,7>)
    n312 = Multiply(x=w573, y=w587) -> (x*y=w581:fxp<+/-,44,14>)
    n313 = Select(t=w574, s=w583, f=fxp<+/-,2,2> 1.0) -> (s? t:f=w568:fxp<+/-,33,2>)
    n314 = Multiply(x=w572, y=w580) -> (x*y=w578:fxp<+/-,38,6>)
    n315 = Multiply(x=w568, y=w581) -> (x*y=w571:fxp<+/-,36,14>)
    "omega_p (Mavg)" <- w571
    n316 = Divide(x=w578, y=w579) -> (x/y=w570:fxp<+/-,45,6>)
    n317 = Multiply(x=w570, y=w571) -> (x*y=→"Dp_d (Mavg)":fxp<+/-,36,14>)
  }
  n318 = while "PID force controller_p" {
    shift-right: [w634] -> _
    shift-left: _ -> [w633]
    stop <- FALSE stop-if-true
    n319 = local read "D_p(mm)"() -> (w628:fxp<+/-,32,7>)
    n320 = local read "Dpr_for"() -> (w629:fxp<+/-,22,7>)
    n321 = call "Tick Count7"() -> ("Tick Count(uSec)"=w634:u32)
    n322 = Subtract(x=w629, y=w628) -> (x-y=w627:fxp<+/-,33,8>)
    n323 = Subtract(x=w634, y=w633) -> (x-y=w632:u32)
    n324 = Multiply(x="Kp_p", y=w627) -> (x*y=→"Fp_PID":fxp<+/-,64,20>)
    n325 = Divide(x=u32 1000, y=w632) -> (x/y=→"PID (kHz)":fxp<+/-,20,7>)
  }
  n326 = while "Quadrature drive_p" {
    stop <- FALSE stop-if-true
    n327 = local read "omega_p (rad/s)"() -> (w642:fxp<+/-,36,13>)
    n328 = local read "Fp_PID"() -> (w638:fxp<+/-,36,16>)
    n329 = call "Oriental_step_motor_PKP225.vi"("F_Threshold"=fxp<+,12,12> 10.0, "dFmr"=fxp<+,1,1> 0.0 ("f"), "omega"=w642, "Fmr"=w638) -> ("vq_F"=→"vq_p_F":fxp<+/-,20,5>, "vd_F"=→"vd_p_F":fxp<+/-,20,5>)  [unwired: 6 in]
  }
  n330 = while "All switch" {
    stop <- FALSE stop-if-true
    n331 = case shown="True" "Encoder reset" {
      frame False {
        n332 = local write "Encoder reset_p"(FALSE ("Encoder reset_p")) -> ()
        n333 = local write "Encoder reset_y"(FALSE ("Encoder reset_y")) -> ()
      }
      frame True {
        n334 = flat-sequence {
          frame #0 {
            n335 = local write "Encoder reset_p"(TRUE ("Encoder reset_p")) -> ()
          }
          frame #1 {
            n336 = local write "Encoder reset_y"(TRUE ("Encoder reset_y")) -> ()
            n337 = local write "Encoder reset_p"(FALSE ("Encoder reset_p")) -> ()
          }
          frame #2 {
            n338 = local write "Encoder reset_y"(FALSE ("Encoder reset_y")) -> ()
          }
        }
      }
    }
  }
  n339 = while "Encoder_y" {
    shift-right: [w689] -> _
    shift-left: _ -> [w681]
    shift-right: [w688] -> _
    shift-left: _ -> [w680]
    shift-right: [w679] -> _
    shift-left: _ -> [w677]
    shift-right: [w685] -> _
    shift-left: _ -> [w682]
    shift-right: [w684] -> _
    shift-left: _ -> [w683]
    shift-right: [w678] -> _
    shift-left: _ -> [w676]
    stop <- FALSE stop-if-true
    w666 = fxp<+/-,16,1> 0.0244140625  # 2*50/4096
    w671 = fxp<+/-,20,-5> 0.00048828125  # L/4096
    w674 = fxp<+/-,20,-5> 0.002499997615814209  # L/800
    w656 = fxp<+/-,16,1> 0.125  # 2*50/800
    n340 = xnode "FPGA I/O Node"() -> ("Mod7/DIO2"=w690:bool, "Mod7/DIO3"=w691:bool)  [unwired: 2 in, 2 out]
    n341 = xnode "FPGA I/O Node"() -> ("Mod7/DIO6"=w687:bool, "Mod7/DIO7"=w686:bool)  [unwired: 2 in, 2 out]
    n342 = local read "Encoder reset_y"() -> (w661:bool)
    n343 = call "encoder_sub.vi"("A_pre"=w681, "B_pre"=w680, "Encoder Position_pre"=w677, "A input"=w690, "Encoder Position Reset"="Encoder reset_y", "B input"=w691) -> ("A"=w689:bool, "B"=w688:bool, "Encoder Position (Counts)"=w679:i32)  [unwired: 19 in]
    "Encoder Position_y1" <- w679
    n344 = call "encoder_sub.vi"("A_pre"=w682, "B_pre"=w683, "Encoder Position_pre"=w676, "A input"=w687, "Encoder Position Reset"=w661, "B input"=w686) -> ("A"=w685:bool, "B"=w684:bool, "Encoder Position (Counts)"=w678:i32)  [unwired: 19 in]
    "Encoder Position_y2" <- w678
    n345 = local read "Belt_in_y"() -> (w669:fxp<+/-,6,6>)
    n346 = local read "Belt_in_y"() -> (w673:fxp<+/-,6,6>)
    n347 = local read "Belt_out_y"() -> (w667:fxp<+/-,7,7>)
    n348 = Divide(x=w671, y="Mag. factor_y") -> (x/y=w670:fxp<+/-,41,13>)
    n349 = local read "Belt_out_y"() -> (w672:fxp<+/-,7,7>)
    n350 = To Fixed-Point(number=w678) -> (fixed-point=w653:fxp<+/-,32,32>)  [unwired: 1 in]
    n351 = local read "Mag. factor_y"() -> (w665:fxp<+/-,20,3>)
    n352 = To Fixed-Point(number=w679) -> (fixed-point=w657:fxp<+/-,32,32>)  [unwired: 1 in]
    n353 = Multiply(x=w670, y=w669) -> (x*y=w668:fxp<+/-,46,18>)
    n354 = Multiply(x=w674, y=w673) -> (x*y=w675:fxp<+/-,26,1>)
    n355 = Divide(x=w668, y=w667) -> (x/y=w655:fxp<+/-,53,18>)
    n356 = Divide(x=w675, y=w672) -> (x/y=w659:fxp<+/-,33,1>)
    n357 = Divide(x=w666, y=w665) -> (x/y=w652:fxp<+/-,32,1>)
    n358 = Multiply(x=w655, y=w653) -> (x*y=→"D_y2":fxp<+/-,37,7>)
    n359 = Multiply(x=w657, y=w656) -> (x*y=→"rad_y1":fxp<+/-,33,20>)
    n360 = Multiply(x=w659, y=w657) -> (x*y=→"D_y1":fxp<+/-,32,7>)
    n361 = Multiply(x=w653, y=w652) -> (x*y=→"rad_y2":fxp<+/-,33,20>)
  }
  n362 = while "Omega_y(T method)" {
    shift-right: [w718] -> _
    shift-left: _ -> [w719]
    shift-right: [w695] -> _
    shift-left: _ -> [w721]
    shift-right: [w723] -> _
    shift-left: _ -> [w724]
    shift-right: [w711] -> _
    shift-left: _ -> [w709]
    shift-right: [w704] -> _
    shift-left: _ -> [w710]
    shift-right: [w707] -> _
    shift-left: _ -> [w708]
    stop <- FALSE stop-if-true
    w702 = fxp<+/-,32,0> 0.3183098859153688  # L/2/pi
    w713 = fxp<+,32,0> 0.1953125  # 800/4096
    w717 = fxp<+/-,32,0> 0.3183098859153688  # L/2/pi
    n363 = local read "Encoder Position_y1"() -> (w718:i32)
    n364 = call "Tick Count2"() -> ("Tick Count(Ticks)"=w705:u32)
    n365 = local read "Encoder Position_y2"() -> (w711:i32)
    n366 = local read "Mag. factor_y"() -> (w712:fxp<+/-,20,3>)
    n367 = call "omega_sub_Encoder_800ppr.vi"("mt0"="mt0_omega_y", "omega_pre"=w721, "ticks_m_pre"=w724, "ticks"=w705, "count_pre"=w719, "count"=w718) -> ("ticks_m"=w723:u32, "mt"=→"mt_omega_y1":u32, "omega"=w695:fxp<+/-,36,13>)  [unwired: 3 in]
    "omega_y1 (T)" <- w695
    n368 = call "omega_sub_Encoder_800ppr.vi"("omega_pre"=w710, "ticks_m_pre"=w708, "ticks"=w705, "count_pre"=w709, "count"=w711) -> ("ticks_m"=w707:u32, "mt"=→"mt_omega_y2":u32, "omega"=w704:fxp<+/-,36,13>)  [unwired: 4 in]
    n369 = local read "Belt_in_y"() -> (w701:fxp<+/-,6,6>)
    n370 = local read "Belt_out_y"() -> (w699:fxp<+/-,7,7>)
    n371 = Divide(x=w713, y=w712) -> (x/y=w703:fxp<+/-,32,1>)
    n372 = Multiply(x=w717, y="Belt_in_y") -> (x*y=w715:fxp<+/-,38,6>)
    n373 = Multiply(x=w702, y=w701) -> (x*y=w700:fxp<+/-,38,6>)
    n374 = Divide(x=w700, y=w699) -> (x/y=w693:fxp<+/-,45,6>)
    n375 = Divide(x=w715, y="Belt_out_y") -> (x/y=w696:fxp<+/-,20,1>)
    n376 = Multiply(x=w704, y=w703) -> (x*y=w692:fxp<+/-,36,13>)
    "omega_y2 (T)" <- w692
    n377 = Multiply(x=w696, y=w695) -> (x*y=→"Dy1_d (T)":fxp<+/-,36,13>)
    n378 = Multiply(x=w693, y=w692) -> (x*y=→"Dy2_d (T)":fxp<+/-,36,13>)
  }
  n379 = while {
    stop <- FALSE stop-if-true
    n380 = local read "omega_p (Mavg)"() -> (w728:fxp<+/-,36,14>)
    n381 = xnode "Butterworth Filter"("input data"=w728, "scaled coefficients"="scaled coefficients") -> ("output data"=→"omega_p (Mavg w. f)":fxp<+/-,36,18>)  [unwired: 1 in]
  }
